vi "Close File.vi"(8 "error in":errorcluster, 11 "File Actor in":refnum<class "File Actor.lvclass">) -> (0 "error out":errorcluster, 3 "File Actor out":refnum<class "File Actor.lvclass">)   [LabVIEW 2014, in "File Library.lvlib" / "File Actor.lvclass"]
doc: "Close the file associated with the object if the current file is valid. If the file only contains a header, then delete the file so that we do not have files propagating for no reason. If the directory is empty after this, delete the directory."
uses:
  File Actor.lvclass
  File Actor.lvclass/File Actor.ctl
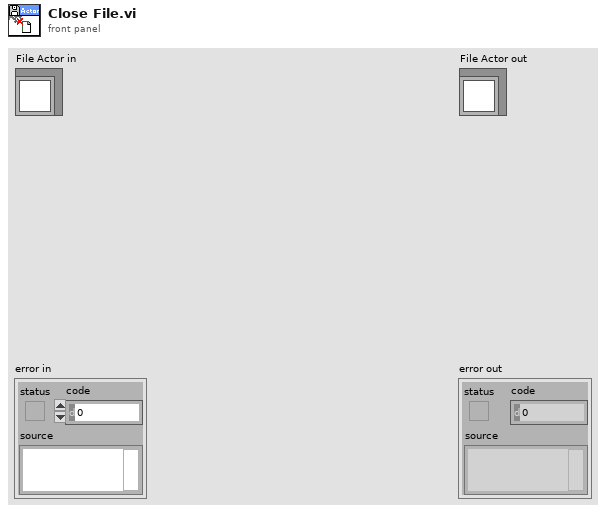
[diagram p1: front panel]
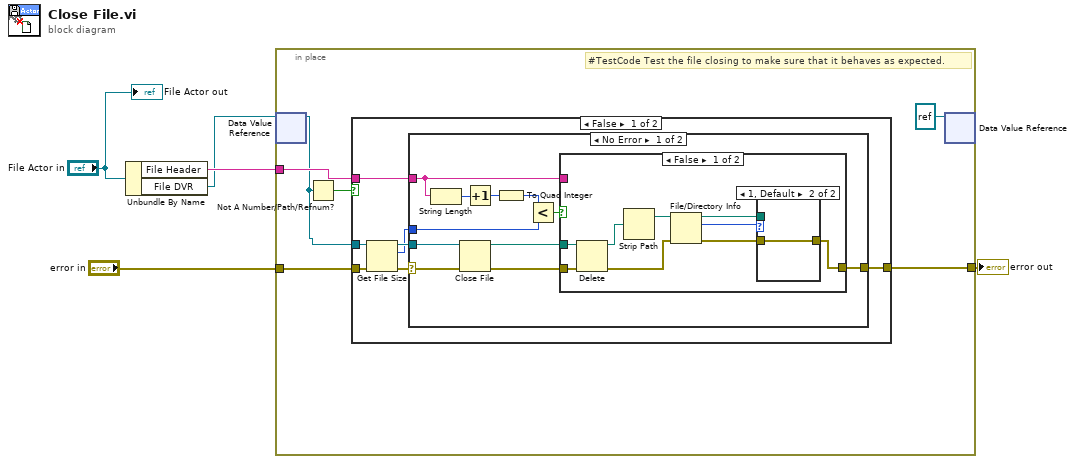
[diagram p0: block diagram]
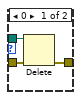
[diagram p2: hidden frame]
diagram:
  n1 = Unbundle By Name("File Actor in") -> ("File Header"=w2:string, "File DVR"=w1:refnum<data-value>)
  n2 = in-place {
    in-place-border: "error in" -> [w10]
    in-place-border: [w9] -> w3
    in-place-border: w2 -> [w8]
    # "#TestCode Test the file closing to make sure that it behaves as expected."
    n3 = in-place-dvr #1(w1) -> (w7:refnum<file>)  [unwired: 1 out]
    n4 = Not A Number/Path/Refnum?(number/path/refnum=w7) -> (NaN/Path/Refnum?=w11:bool)
    n5 = case shown="False" w11 {
      tunnel: w10 -> [w18 w45]
      tunnel: [w17 w45] -> w9
      tunnel: w7 -> [w13 _]
      tunnel: w8 -> [w12 _]
      frame False {
        n6 = Get File Size(file=w13, error in=w18) -> (refnum out=w16:refnum<file>, size (in bytes)=w15:i64, 0:w14:errorcluster)
        n7 = case shown="No Error" w14 {
          selector: w14 -> [w25 w44]
          tunnel: [w29 w44] -> w17
          tunnel: w16 -> [w28 _]
          tunnel: w15 -> [w20 _]
          tunnel: w12 -> [w21 _]
          frame No Error {
            n8 = String Length(string=w21) -> (length=w22:i32)
            n9 = Close File(refnum=w28, error in=w25) -> (path=w26:path, error out=w27:errorcluster)
            n10 = Increment(x=w22) -> (x+1=w23:i32)
            n11 = To Quad Integer(1:w23) -> (0:w24:i64)
            n12 = Less?(x=w24, y=w20) -> (x < y?=w19:bool)
            n13 = case shown="False" w19 {
              tunnel: w27 -> [w38 w43]
              tunnel: w26 -> [w37 _]
              tunnel: [w31 w43] -> w29
              tunnel: w21 -> [_ _]
              frame False {
                n14 = Delete(path (use dialog)=w37, error in=w38) -> (deleted path=w36:path, error out=w32:errorcluster)  [unwired: 3 in, 1 out]
                n15 = Strip Path(path=w36) -> (stripped path=w35:path)  [unwired: 1 out]
                n16 = File/Directory Info(path=w35, error in=w32) -> (path out=w33:path, size=w30:i64, error out=w34:errorcluster)  [unwired: 4 out]
                n17 = case shown="1, Default" w30 {
                  tunnel: w34 -> [w41 w42]
                  tunnel: w33 -> [w40 _]
                  tunnel: [w39 w42] -> w31
                  frame 0 {
                    n18 = Delete(path (use dialog)=w40, error in=w41) -> (error out=w39:errorcluster)  [unwired: 3 in, 2 out]
                  }
                  frame 1, Default {
                  }
                }
              }
              frame True {
              }
            }
          }
          frame Error {
          }
        }
      }
      frame True {
      }
    }
    n19 = in-place-dvr #1(refnum<file> refnum ("data value")) -> ()  [unwired: 2 out]
  }
  "error out" <- w3
  "File Actor out" <- "File Actor in"
